vi "MI.PrependLength.vi"(1 "Command":string) -> (0 "0#Command":string)   [LabVIEW 2016, in "instrument.Cryostation.lvclass"]
uses:
  instrument.Cryostation.lvclass
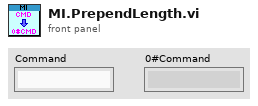
[diagram p1: front panel]
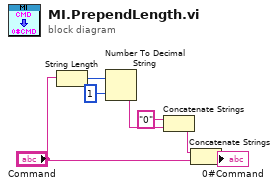
[diagram p0: block diagram]
diagram:
  n1 = String Length(string="Command") -> (length=w1:i32)
  n2 = Number To Decimal String(number=w1, width (-)=i16 1) -> (decimal integer string=w4:string)
  n3 = Concatenate Strings("0" ("string"), w4) -> (w7:string)
  n4 = Concatenate Strings(w7, "Command") -> (→"0#Command":string)
